vi "Control - Diesel - EGR Flow.vi"() -> ()   [LabVIEW 2015, in "ECS-Host.lvlib"]
uses:
  ECS-Host.lvlib
  <vilib>/addons/Software Calibration Management/XControls/TBL2D.xctl
panel:
  out "EGRMassFlow_Calc":sgl caption="[]"
  in  "EGRValveCd_Tbl":cluster{"X":sgl[], "Y":sgl[], "Z":sgl[][]}(xcontrol) caption="[]"
  out "EGRValveCd_TblOut":sgl caption="[]"
  in  "ExhGasRConst":sgl caption="[]"
  in  "ExhGasKConst":sgl caption="[]"
  in  "EGRValveDiameter":sgl caption="[]"
  # "Note:  Requires Exhaust Manifold Pressure, Temperature, and EGR Valve Differential Pressure"
  # "Pressure \nRatio"
  # "EGR Valve Position"
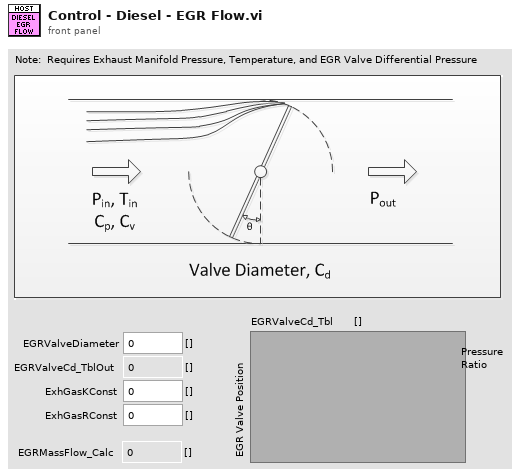
[diagram p1: front panel]
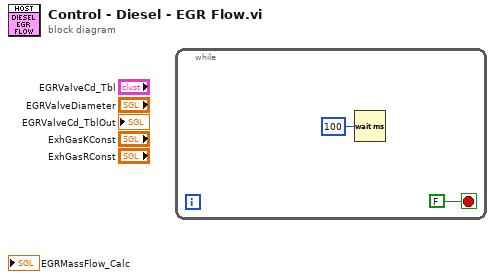
[diagram p0: block diagram]
diagram:
  n1 = while {
    stop <- FALSE stop-if-true
    n2 = Wait (ms)(milliseconds to wait=u32 100) -> ()  [unwired: 1 out]
  }
